vi "filtro Adaptativo LV ECG por TR.vi"() -> ()   [LabVIEW 2014]
doc: "This example demonstrates how to extract fetal electrocardiogram (ECG) signals from maternal abdominal ECG signals. You obtain maternal abdominal ECG signals from obdominal leads. Maternal abdominal ECG signals contain both maternal ECG signals and fetal ECG signals. You can use an adaptive filter to extract fetal ECG signals from maternal abdominal ECG signals. To use an adaptive filter as the solution, you must obtain maternal thorax ECG signals from thorax leads as reference signals."
uses:
  Documents/sd_2015_2/Control 1.ctl
  <vilib>/sound/lvsound.llb/Sound Format.ctl
  <vilib>/addons/Adaptive Filters/Create/AFT Create FIR LMS (Real).vi
  <vilib>/addons/Adaptive Filters/Processing/AFT Filter Signal and Update Coefficients (Real, Array).vi
  <vilib>/addons/Adaptive Filters/NI_AdaptiveFilter.lvlib
  <vilib>/Analysis/NI_AALBase.lvlib
panel:
  in  "stop":bool
  in  "sound format":T1
  in  "Step Size":T2=0.45 min=0.0 step=0.01 format="%#_9f"
  in  "Filter Length":i32=40 min=2
  out "Fetal ECG":dbl[](graph)
  out "Waveform Graph 3":u8[](graph)
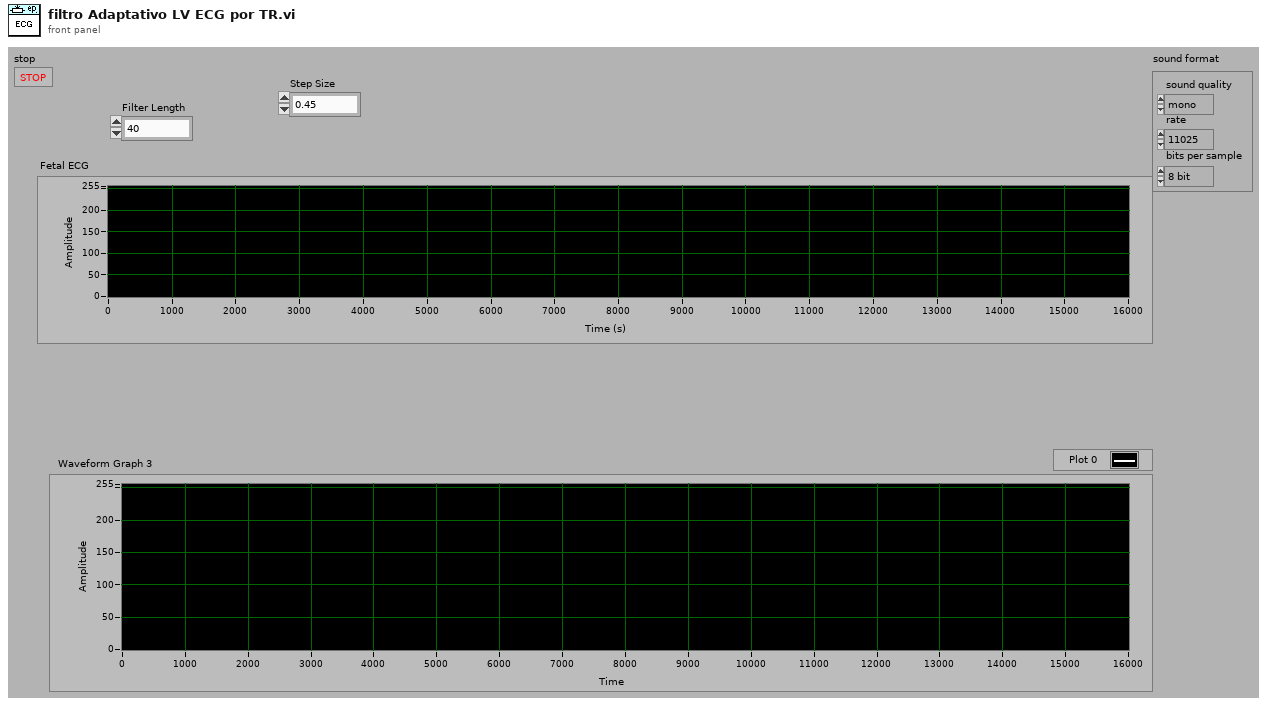
[diagram p1: front panel]
types:
  T1 = typedef "Sound Format.ctl" = cluster{"sound quality":enum16{"mono", "stereo"}, "rate":enum16{"11025", "22050", "44100", "8000"}, "bits per sample":enum16{"8 bit", "16 bit"}}
  T2 = typedef "Control 1.ctl" = dbl
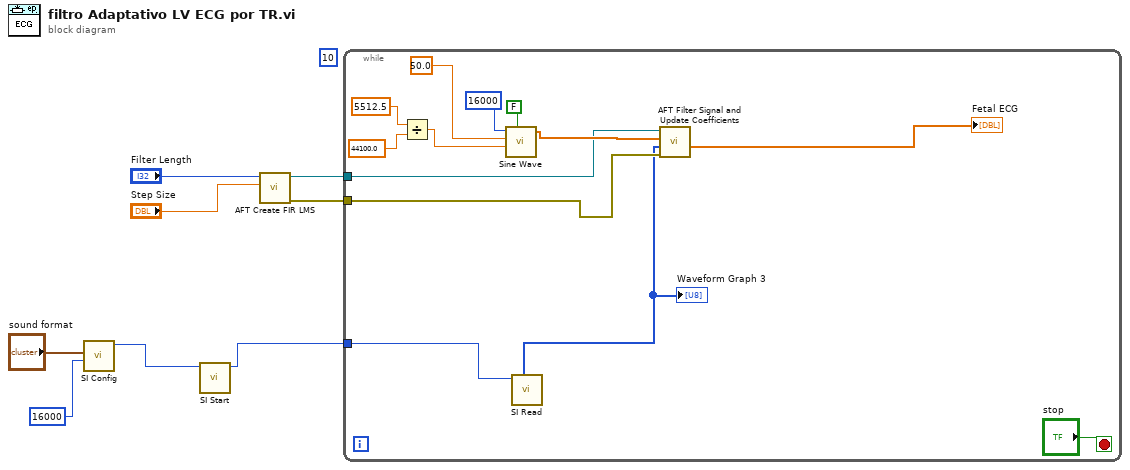
[diagram p0: block diagram]
diagram:
  (unwired) 10
  n1 = call "SI Config.vi"("buffer size (8192 in bytes)"=u32 16000, "sound format"="sound format") -> ("task ID out"=w2:u32)  [unwired: 8 in, 1 out]
  n2 = call "SI Start.vi"("task ID in"=w2) -> ("task ID out"=w1:u32)  [unwired: 9 in, 1 out]
  n3 = call-poly <vilib>:"AFT Create FIR LMS.vi"("step size"="Step Size", "filter length"="Filter Length") -> ("error out"=w5:errorcluster, "adaptive filter out"=w6:refnum<k20>)  [unwired: 2 in, 6 out]
  n4 = while {
    tunnel: w6 -> [w13]
    tunnel: w5 -> [w12]
    tunnel: w1 -> [w11]
    stop <- "stop" stop-if-true
    n5 = Divide(x=5512.5, y=44100.0) -> (x/y=w18:dbl)
    n6 = call <vilib>:"Sine Wave.vi"("samples"=16000, "amplitude"=50.0, "frequency"=w18, "reset phase"=FALSE) -> ("sine wave"=w16:dbl[])  [unwired: 1 in, 2 out]
    n7 = call "SI Read.vi"("task ID in"=w11) -> ("mono 8-bit"=w9:u8[])  [unwired: 5 in, 5 out]
    "Waveform Graph 3" <- w9
    n8 = call-poly <vilib>:"AFT Filter Signal and Update Coefficients.vi"("error in (no error)"=w12, "d(n)"=w9, "x(n)"=w16, "adaptive filter in"=w13) -> ("e(n)"=→"Fetal ECG":dbl[])  [unwired: 2 in, 5 out]
  }
